vi "getColHdrs.vi"(8 "error in (no error)":errorcluster, 11 "DataHandler in":refnum<class "DataHandlerMYiTOPS.lvclass">) -> (0 "error out":errorcluster, 2 "List of ColHads":string[](array[string]), 3 "DataHandler out":refnum<class "DataHandlerMYiTOPS.lvclass">)   [LabVIEW 2015, in "DataHandlerMYiTOPS.lvclass"]
uses:
  DataHandlerMYiTOPS.lvclass
  <vilib>/regexp/Match Regular Expression.xnode
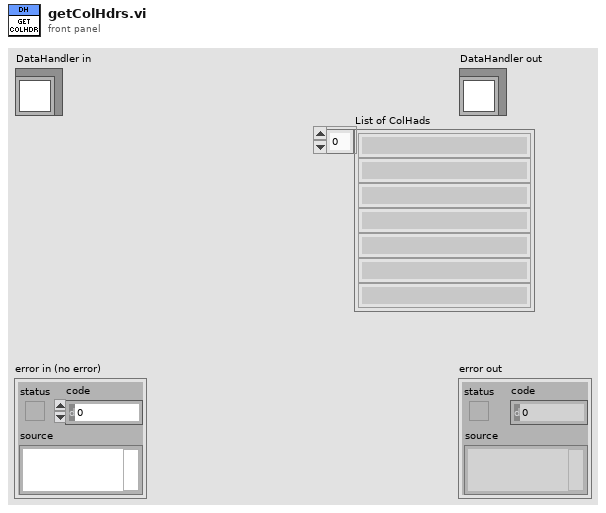
[diagram p1: front panel]
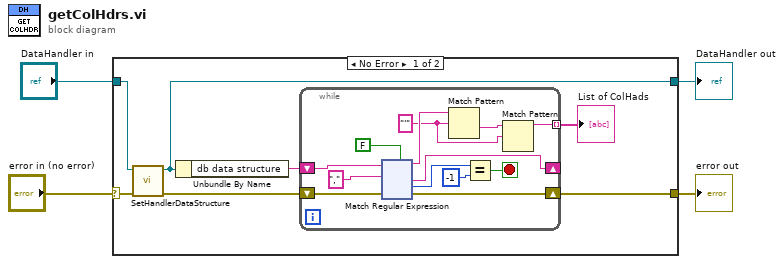
[diagram p0: block diagram]
diagram:
  n1 = case shown="No Error" "error in (no error)" {
    selector: "error in (no error)" -> [w10 w140]
    tunnel: [w5 w140] -> w3
    tunnel: [w9 w139] -> w1
    tunnel: "DataHandler in" -> [w11 w139]
    frame No Error {
      n2 = call-dynamic "SetHandlerDataStructure.vi"("error in (no error)"=w10, "DataHandler in"=w11) -> ("error out"=w6:errorcluster, "DataHandler out"=w9:refnum<class "DataHandlerMYiTOPS.lvclass">)  [unwired: 8 in]
      n3 = Unbundle By Name(w9) -> ("db data structure"=w8:string)
      n4 = while {
        shift-right: [w22] -> _
        shift-left: w8 -> [w23]
        tunnel: [w13] -> w7 mode=indexing
        shift-right: [w16] -> w5
        shift-left: w6 -> [w17]
        stop <- w18 stop-if-true
        w12 = "'" ("regular expression")
        n5 = xnode "Match Regular Expression"("input string"=w23, "regular expression"=",", "error in"=w17, "multiline? (F)"=FALSE) -> ("before match"=w15:string, "after match"=w22:string, "offset past match"=w20:i32, "error out"=w16:errorcluster)  [unwired: 2 in, 1 out]
        n6 = Match Pattern(string=w15, regular expression=w12) -> (after substring=w14:string)  [unwired: 1 in, 3 out]
        n7 = Equal?(x=w20, y=-1) -> (x = y?=w18:bool)
        n8 = Match Pattern(string=w14, regular expression=w12) -> (before substring=w13:string)  [unwired: 1 in, 3 out]
      }
      "List of ColHads" <- w7
    }
    frame Error {
    }
  }
  "error out" <- w3
  "DataHandler out" <- w1
